vi "Pull_Data_via_Public_Server.vi"(0 "Path of File relative to EnFlo Data Root":path[](array[path])) -> (2 "Relative Paths Out":path[](array[path]), 3 "Problem Files":path[](array[path]), 4 "error out":errorcluster)   [LabVIEW 2016]
uses:
  Anemometry/Anemometry Sub Vis/Globals/Constants_global.vi
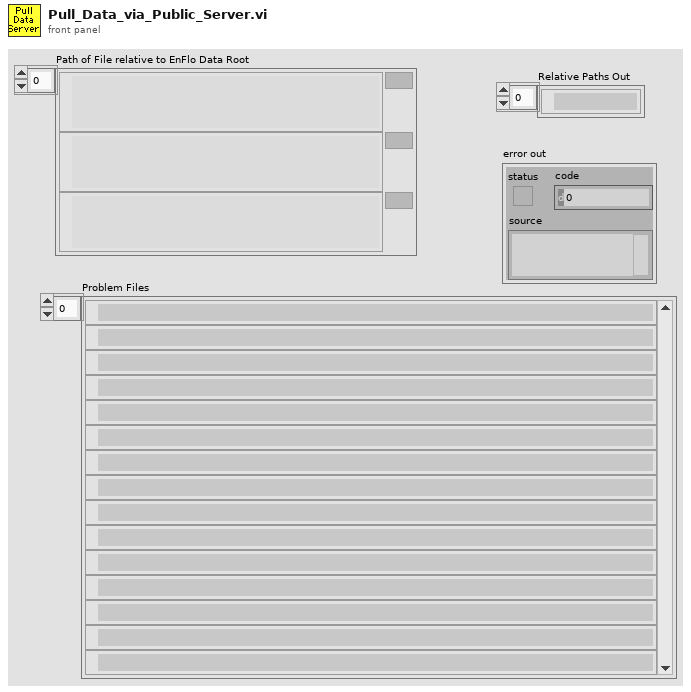
[diagram p1: front panel]
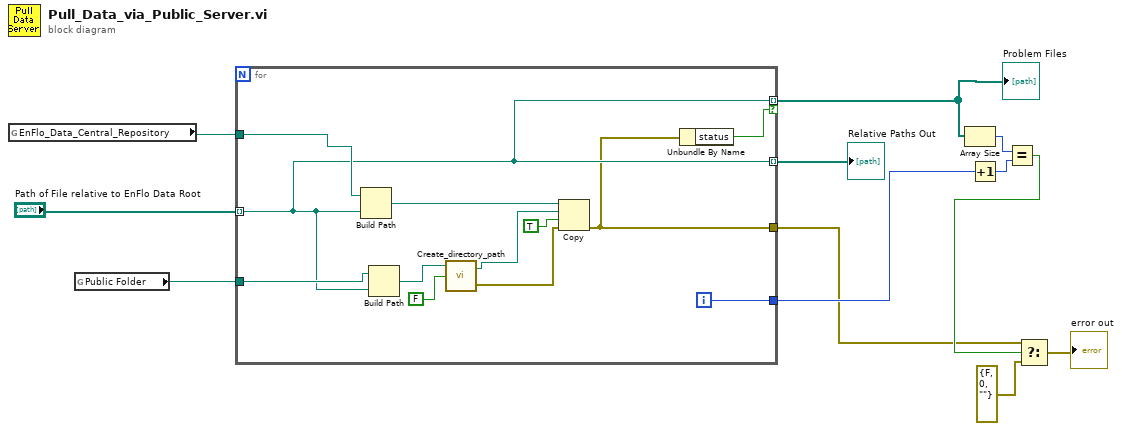
[diagram p0: block diagram]
diagram:
  n1 = global read "Constants_global.vi" "EnFlo_Data_Central_Repository"() -> (w12:path)
  n2 = global read "Constants_global.vi" "Public Folder"() -> (w10:path)
  n3 = for {
    tunnel: w12 -> [w24]
    tunnel: "Path of File relative to EnFlo Data Root" -> [w16] mode=indexing
    tunnel: w10 -> [w23]
    tunnel: [w15] -> w2
    tunnel: [w16] -> w9 mode=indexing
    tunnel: [w16] -> w4 mode=indexing if=w14
    tunnel: [w13] -> w3
    i -> [w13]
    n4 = Build Path(base path=w24, name or relative path=w16) -> (appended path=w21:path)
    n5 = Build Path(base path=w23, name or relative path=w16) -> (appended path=w22:path)
    n6 = call "Create_directory_path.vi"("Dialog Box"=FALSE, "Path name"=w22) -> ("error out"=w19:errorcluster, "Path name Out"=w20:path)  [unwired: 1 in]
    n7 = Copy(8:w19, 9:TRUE ("overwrite (F)"), 10:w20, 11:w21) -> (0:w15:errorcluster)  [unwired: 1 in, 2 out]
    n8 = Unbundle By Name(w15) -> ("status"=w14:bool)
  }
  "Relative Paths Out" <- w9
  "Problem Files" <- w4
  n9 = Array Size(array=w4) -> (size(s)=w5:i32)
  n10 = Increment(x=w3) -> (x+1=w6:i32)
  n11 = Equal?(x=w5, y=w6) -> (x = y?=w7:bool)
  n12 = Select(t=w2, s=w7, f=errorcluster {"status"=FALSE, "code"=0, "source"=""} ("error out")) -> (s? t:f=→"error out":errorcluster)
